vi "GetAnalog.vi"(7 "Port Distant":u16, 8 "entrée d'erreur (pas d'erreur)":errorcluster, 9 "Adresse IP":u32, 10 "Pin":u8, 11 "Connexion réseau UDP en entrée":refnum<k16>) -> (0 "sortie d'erreur":errorcluster, 2 "Return Value":u16, 3 "Connexion réseau UDP en sortie":refnum<k16>)   [LabVIEW 2021]
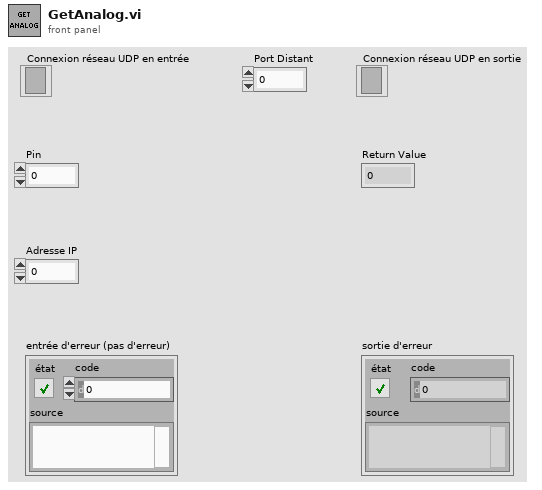
[diagram p1: front panel]
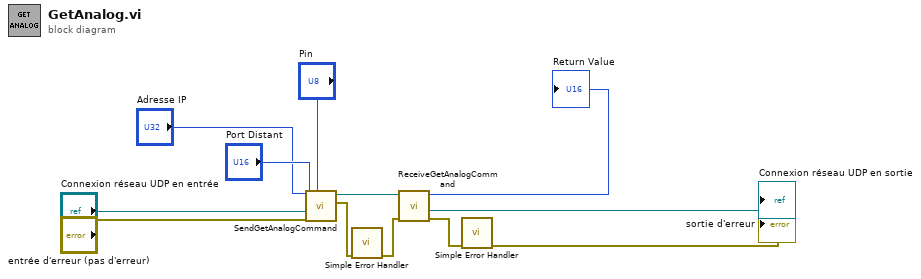
[diagram p0: block diagram]
diagram:
  n1 = call "SendGetAnalogCommand.vi"("Pin"="Pin", "entrée d'erreur"="entrée d'erreur (pas d'erreur)", "Port Destination"="Port Distant", "Adresse IP Destination"="Adresse IP", "Connexion réseau UDP en entrée"="Connexion réseau UDP en entrée") -> ("sortie d'erreur 2"=w8:errorcluster, "Connexion réseau UDP en sortie"=w6:refnum<k16>)  [unwired: 5 in]
  n2 = call <vilib>:"Simple Error Handler.vi"("error in (no error)"=w8) -> ("error out"=w9:errorcluster)  [unwired: 4 in, 4 out]
  n3 = call "ReceiveGetAnalogCommand.vi"("entrée d'erreur (pas d'erreur)"=w9, "Connexion réseau UDP en entrée"=w6) -> ("sortie d'erreur"=w10:errorcluster, "Connexion réseau UDP en sortie"=→"Connexion réseau UDP en sortie":refnum<k16>, "Numérique"=→"Return Value":u16)  [unwired: 6 in, 1 out]
  n4 = call <vilib>:"Simple Error Handler.vi"("error in (no error)"=w10) -> ("error out"=→"sortie d'erreur":errorcluster)  [unwired: 4 in, 4 out]
